vi "sendAckNoAckToClient.vi"(8 "error in (no error)":errorcluster, 9 "ackIterations":i32, 10 "packetConnID":T1, 11 "tcpServer in":refnum<class "TcpServer.lvclass">) -> (0 "error out":errorcluster, 2 "packetConnID":T1, 3 "tcpServer out":refnum<class "TcpServer.lvclass">)   [LabVIEW 2018, in "TcpServer.lvclass"]
doc: "Send the ack to the TCP Client for the last command received, and if there are lost commands, it sends noAck for them."
uses:
  TcpServer.lvclass
  typedef/packetConnIDTypeDef.ctl
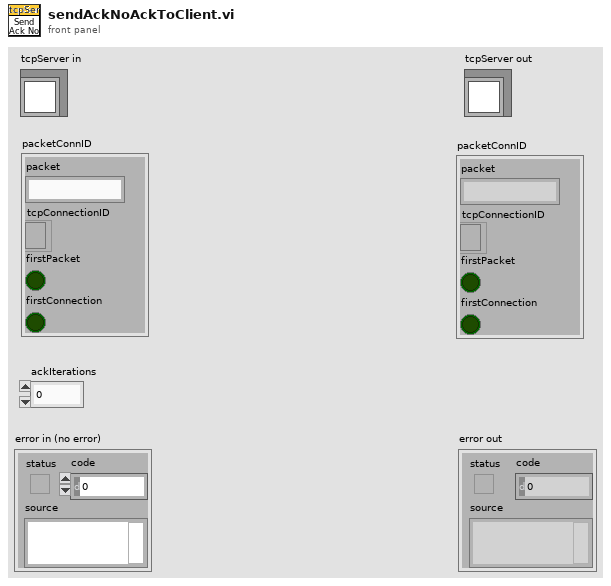
[diagram p1: front panel]
types:
  T1 = typedef "TcpServer.lvclass/packetConnIDTypeDef.ctl" = cluster{"packet":string, "tcpConnectionID":refnum<k5>, "firstPacket":bool, "firstConnection":bool}
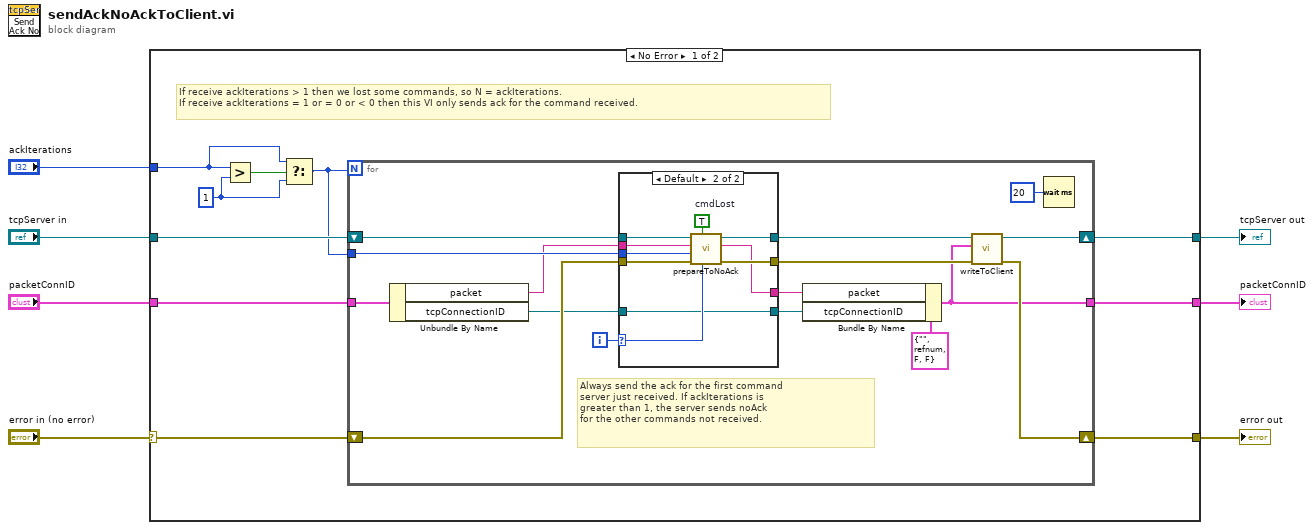
[diagram p0: block diagram]
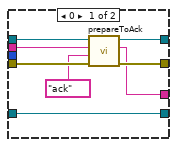
[diagram p2: hidden frame]
diagram:
  n1 = case shown="No Error" "error in (no error)" {
    selector: "error in (no error)" -> [w17 w52]
    tunnel: [w16 w52] -> w6
    tunnel: "tcpServer in" -> [w15 w54]
    tunnel: [w14 w54] -> w4
    tunnel: "packetConnID" -> [w13 w53]
    tunnel: [w12 w53] -> w2
    tunnel: "ackIterations" -> [w10 _]
    frame No Error {
      w9 = 1 ("y")
      # "If receive ackIterations > 1 then we lost some commands, so N = ackIterations.\nIf receive ackIterations = 1 or = 0 or < 0 then this VI only sends ack for the command received."
      n2 = Greater?(x=w10, y=w9) -> (0:w11:bool)
      n3 = Select(t=w10, s=w11, f=w9) -> (s? t:f=w8:i32)
      n4 = for {
        N: w8 -> [_]
        tunnel: w13 -> [w29]
        tunnel: w8 -> [w28]
        shift-right: [w32] -> w16
        shift-left: w17 -> [w33]
        shift-right: [w30] -> w14
        shift-left: w15 -> [w31]
        tunnel: [w18] -> w12
        i -> [w21]
        # "Always send the ack for the first command\nserver just received. If ackIterations is \ngreater than 1, the server sends noAck \nfor the other commands not received."
        n5 = Unbundle By Name(w29) -> ("packet"=w25:string, "tcpConnectionID"=w19:refnum<k5>)
        n6 = case shown="Default" w21 {
          selector: w21 -> [_ w44]
          tunnel: w33 -> [w38 w51]
          tunnel: w31 -> [w40 w50]
          tunnel: w28 -> [_ w49]
          tunnel: [w39 w48] -> w27
          tunnel: [w37 w47] -> w26
          tunnel: w25 -> [w36 w46]
          tunnel: [w34 w45] -> w23
          tunnel: [w41 w43] -> w20
          tunnel: w19 -> [w41 w43]
          frame 0 {
            n7 = call "prepareToAck.vi"("error in (no error)"=w38, "cmdStatus"="ack", "cmd"=w36, "TcpServer in"=w40) -> ("error out"=w37:errorcluster, "JSON string"=w34:string, "TcpServer out"=w39:refnum<class "TcpServer.lvclass">)  [unwired: 5 in]
          }
          frame Default {
            w42 = TRUE  # cmdLost
            n8 = call "prepareToNoAck.vi"("iteration"=w44, "cmdLost"=w42, "error in (no error)"=w51, "lostCmdId"=w49, "cmd"=w46, "TcpServer in"=w50) -> ("error out"=w47:errorcluster, "JSON string"=w45:string, "TcpServer out"=w48:refnum<class "TcpServer.lvclass">)  [unwired: 3 in]
          }
        }
        n9 = Bundle By Name(cluster=T1 {"packet"="", "tcpConnectionID"=refnum, "firstPacket"=FALSE, "firstConnection"=FALSE} ("packetConnID"), "packet"=w23, "tcpConnectionID"=w20) -> (w18:T1)
        n10 = call "writeToClient.vi"("error in (no error)"=w26, "packetConnID"=w18, "tcpServer in"=w27) -> ("error out"=w32:errorcluster, "tcpServer out"=w30:refnum<class "TcpServer.lvclass">)  [unwired: 7 in]
        n11 = Wait (ms)(milliseconds to wait=u32 20) -> ()  [unwired: 1 out]
      }
    }
    frame Error {
    }
  }
  "error out" <- w6
  "tcpServer out" <- w4
  "packetConnID" <- w2
